vi "DIAdem Report Wizard Ole Calls CSB.vi"(8 "error in (no error)":errorcluster, 10 "Source Definition (XML Syntax)":string, 11 "Data File (Path and File)":path) -> (0 "error out":errorcluster)   [LabVIEW 2020]
doc: "This VI uses the DIAdem OLE mechanism to load a layout using the Report Wizard mechanism without launching the wizard dialog."
uses:
  <vilib>/ExportToExcel/Window Modes.ctl
  <vilib>/ExportToExcel/Window Names.ctl
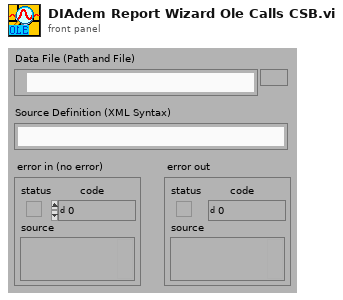
[diagram p1: front panel]
types:
  T1 = typedef "Window Modes.ctl" = enum16{"OPEN", "CLOSE", "SHOW", "MAXIMIZE", "MINIMIZE", "NORMAL", "FULLSIZE"}
  T2 = typedef "DIAdem Reference.ctl" = cluster{"ToCommand Reference":refnum<k7>, "ToDataSheet Reference":refnum<k7>}
  T3 = typedef "Window Names.ctl" = u16
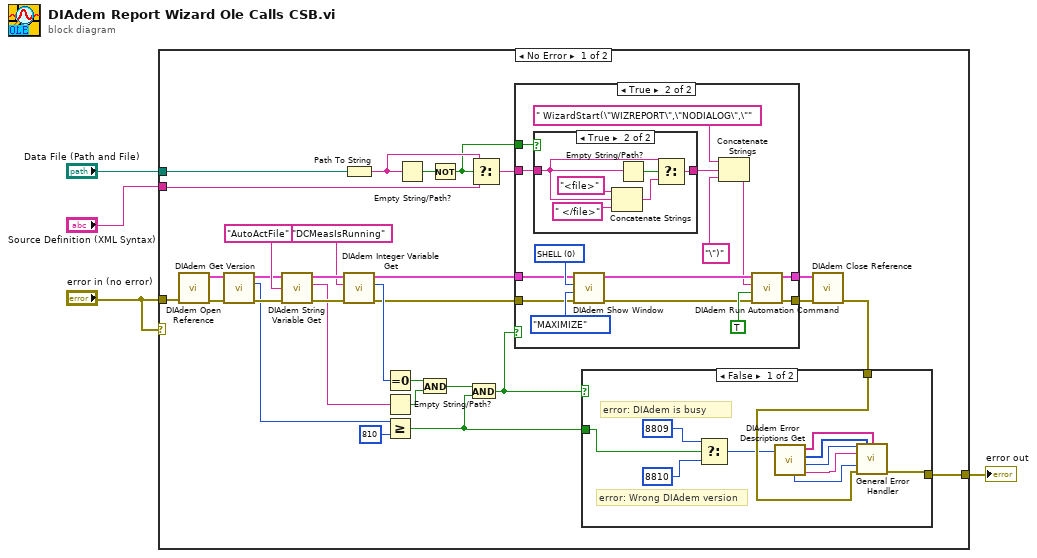
[diagram p0: block diagram]
diagram:
  n1 = case shown="No Error" "error in (no error)" {
    tunnel: "error in (no error)" -> [w18 w71]
    tunnel: "Data File (Path and File)" -> [w17 _]
    tunnel: [w5 w71] -> w3
    tunnel: "Source Definition (XML Syntax)" -> [w14 _]
    frame No Error {
      n2 = call <vilib>:"DIAdem Open Reference.vi"("error in (no error)"=w18) -> ("error out"=w33:errorcluster, "DIAdem Reference"=w32:T2)  [unwired: 9 in]
      n3 = call <vilib>:"DIAdem Get Version.vi"("error in (no error)"=w33, "DIAdem Reference"=w32) -> ("error out"=w23:errorcluster, "Revision"=w21:i32, "DIAdem Reference"=w31:T2)  [unwired: 5 in, 1 out]
      n4 = call <vilib>:"DIAdem String Variable Get.vi"("error in (no error)"=w23, "Variable Name"="AutoActFile" ("command"), "DIAdem Reference"=w31) -> ("error out"=w24:errorcluster, "Value"=w10:string, "DIAdem Reference"=w28:T2)  [unwired: 6 in]
      n5 = Path To String(path=w17) -> (string=w13:string)
      n6 = call <vilib>:"DIAdem Integer Variable Get.vi"("error in (no error)"=w24, "Variable Name"="DCMeasIsRunning", "DIAdem Reference"=w28) -> ("error out"=w22:errorcluster, "Value"=w25:i32, "DIAdem Reference"=w27:T2)  [unwired: 6 in]
      n7 = Equal To 0?(x=w25) -> (x = 0?=w19:bool)
      n8 = Empty String/Path?(string/path=w10) -> (empty?=w9:bool)
      n9 = Greater Or Equal?(x=w21, y=810 ("Revision")) -> (x >= y?=w7:bool)
      n10 = Empty String/Path?(string/path=w13) -> (empty?=w15:bool)
      n11 = And(x=w19, y=w9) -> (x .and. y?=w11:bool)
      n12 = Not(x=w15) -> (.not. x?=w12:bool)
      n13 = And(x=w11, y=w7) -> (x .and. y?=w6:bool)
      n14 = Select(t=w13, s=w12, f=w14) -> (s? t:f=w16:string)
      n15 = case shown="True" w6 {
        tunnel: w22 -> [w48 w60]
        tunnel: [w48 w58] -> w30
        tunnel: w27 -> [w47 w61]
        tunnel: [w47 w59] -> w29
        tunnel: w16 -> [_ w50]
        tunnel: w12 -> [_ w51]
        frame False {
        }
        frame True {
          w62 = T3 0 items=["SHELL", "NAVIGATOR", "ANALYSIS", "REPORT", "VIEW", "VISUAL", "DAC"] ("Window")
          n16 = case shown="True" w51 {
            tunnel: w50 -> [w64 w66]
            tunnel: [w64 w65] -> w49
            frame False {
            }
            frame True {
              n17 = Concatenate Strings("<file>" ("Substring"), w66, " </file>" ("Substring")) -> (w67:string)
              n18 = Empty String/Path?(string/path=w66) -> (empty?=w70:bool)
              n19 = Select(t=w66, s=w70, f=w67) -> (s? t:f=w65:string)
            }
          }
          n20 = call <vilib>:"DIAdem Show Window.vi"("error in (no error)"=w60, "mode"=Window_Modes."MAXIMIZE" ("Mode"), "window"=w62, "DIAdem Reference"=w61) -> ("error out"=w56:errorcluster, "DIAdem Reference"=w55:T2)  [unwired: 6 in]
          n21 = Concatenate Strings(" WizardStart(\"WIZREPORT\",\"NODIALOG\",\"" ("command"), w49, "\")" ("Substring")) -> (w52:string)
          n22 = call <vilib>:"DIAdem Run Automation Command.vi"("error in (no error)"=w56, "asynchronous? (F)"=TRUE, "command"=w52, "DIAdem Reference"=w55) -> ("error out"=w58:errorcluster, "DIAdem Reference"=w59:T2)  [unwired: 6 in]
        }
      }
      n23 = call <vilib>:"DIAdem Close Reference.vi"("error in (no error)"=w30, "DIAdem Reference"=w29) -> ("error out"=w8:errorcluster)  [unwired: 9 in]
      n24 = case shown="False" w6 {
        tunnel: w8 -> [w40 w46]
        tunnel: [w39 w46] -> w5
        tunnel: w7 -> [w35 _]
        frame False {
          # "error: Wrong DIAdem version"
          # "error: DIAdem is busy"
          n25 = Select(t=8809 ("[error code] (0)"), s=w35, f=8810 ("[error code] (0)")) -> (s? t:f=w38:i32)
          n26 = call <vilib>:"DIAdem Error Descriptions Get.vi"("internal error code"=w38) -> ("error source"=w42:string, "error code"=w43:i32, "DIAdem error codes"=w44:i32[], "DIAdem error descriptions"=w45:string[], "type of dialog"=w41:u16)  [unwired: 5 in, 1 out]
          n27 = call <vilib>:"General Error Handler.vi"("[error code] (0)"=w43, "[user-defined codes]"=w44, "[user-defined descriptions]"=w45, "[error source] (\" \")"=w42, "type of dialog (OK msg:1)"=w41, "error in (no error)"=w40) -> ("error out"=w39:errorcluster)  [unwired: 5 in, 4 out]
        }
        frame True {
        }
      }
    }
    frame Error {
    }
  }
  "error out" <- w3
